vi "Data_Array_test.vi"() -> ()   [LabVIEW 2021]
uses:
  Data_Array.lvclass
panel:
  out "Index":i32
  out "Waveform Graph":dbl[](graph)
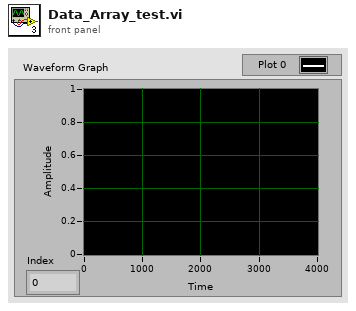
[diagram p1: front panel]
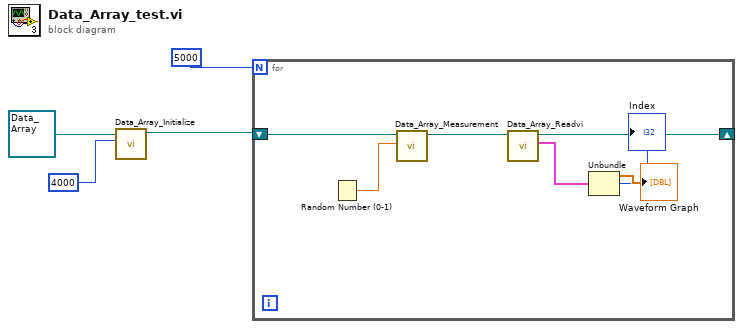
[diagram p0: block diagram]
diagram:
  n1 = call-dynamic "Data_Array_Initialize.vi"("Buffer"=4000, "Data_Array in"=refnum<class "Data_Array.lvclass"> refnum ("Data_Array.lvclass")) -> ("Data_Array out"=w3:refnum<class "Data_Array.lvclass">)  [unwired: 8 in, 1 out]
  n2 = for {
    N: 5000 -> [_]
    shift-right: [w8] -> _
    shift-left: w3 -> [w11]
    n3 = Random Number (0-1)() -> (number: 0 to 1=w10:dbl)
    n4 = call-dynamic "Data_Array_Measurement.vi"("Measurement"=w10, "Data_Array in"=w11) -> ("Data_Array out"=w9:refnum<class "Data_Array.lvclass">)  [unwired: 8 in, 1 out]
    n5 = call-dynamic "Data_Array_Readvi.vi"("Data_Array in"=w9) -> ("Data_params"=w7:cluster{"Data":dbl[], "Index":i32, "Buffer":i32}, "Data_Array out"=w8:refnum<class "Data_Array.lvclass">)  [unwired: 8 in, 1 out]
    n6 = Unbundle(w7) -> ("Data"=→"Waveform Graph":dbl[], "Index"=→"Index":i32)  [unwired: 1 out]
  }
